vi "Find and Disable Selected Opposing Channels.vi"(8 "error in (no error)":errorcluster, 9 "Parent":string, 10 "Item Ref in":T1 format="%.0x", 11 "Tree":refnum<vi>) -> (0 "error out":errorcluster, 2 "Item Ref out":T1 format="%.0x", 3 "Tree Out":refnum<vi>)   [LabVIEW 2013, in "J1939 Addon System Explorer.lvlib"]
uses:
  J1939 Addon System Explorer.lvlib
  <vilib>/NI Veristand/Custom Device API/Custom Device Item Ref.ctl
  <vilib>/NI Veristand/Custom Device Tools/Custom Device Utility Library/Search Direction.ctl
  Shared/SubVIs/Constants.vi
  <vilib>/NI Veristand/Custom Device Tools/Custom Device Utility Library/Custom Device Utility Library.lvlib
  Shared/J1939 Addon Shared.lvlib
  <vilib>/NI Veristand/Custom Device API/Custom Device API.lvlib
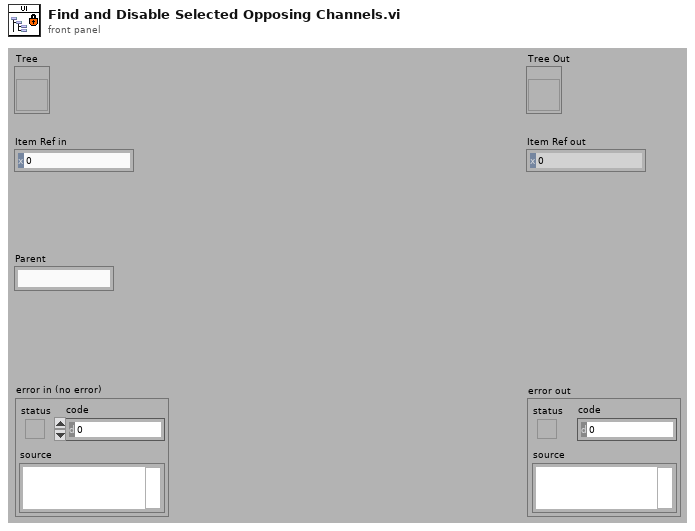
[diagram p1: front panel]
types:
  T1 = typedef "Custom Device API.lvlib/Custom Device Item Ref.ctl" = u64
  T2 = typedef "Custom Device Utility Library.lvlib/Search Direction.ctl" = enum16{"Down", "Up"}
  T3 = typedef "Custom Device API.lvlib/Custom Device Item Info.ctl" = cluster{"Name":string, "Is Channel":bool, "GUID":string, "Is Waveform":bool}
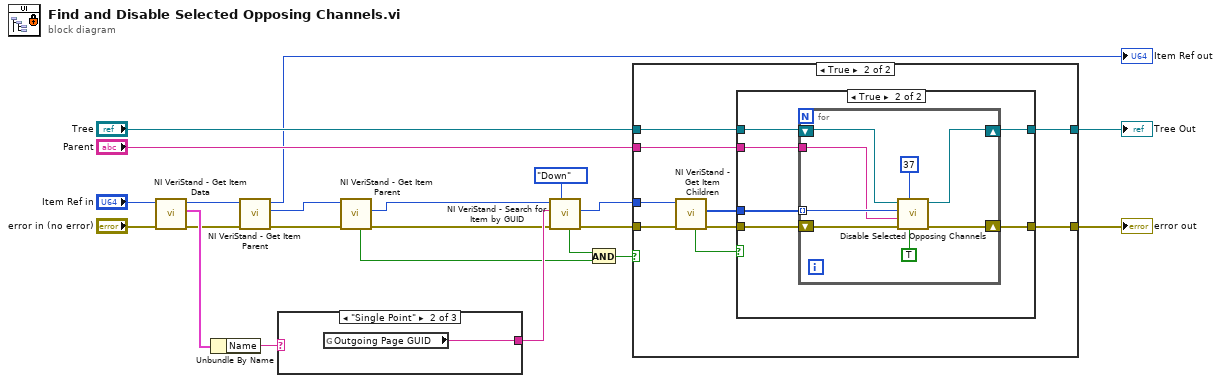
[diagram p0: block diagram]
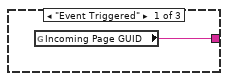
[diagram p4: hidden frame]
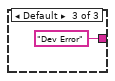
[diagram p5: hidden frame]
diagram:
  n1 = call <vilib>:"NI VeriStand - Get Item Data.vi"("error in (no error)"="error in (no error)", "Item Ref in"="Item Ref in") -> ("error out"=w8:errorcluster, "Item Info"=w21:T3, "Item Ref out"=w7:T1)  [unwired: 7 out]
  n2 = Unbundle By Name(w21) -> ("Name"=w22:string)
  n3 = call <vilib>:"NI VeriStand - Get Item Parent.vi"("error in (no error)"=w8, "Item Ref in"=w7) -> ("error out"=w6:errorcluster, "Parent Ref"=w5:T1, "Item Ref out"=→"Item Ref out":T1)  [unwired: 6 in, 1 out]
  n4 = case shown="\"Single Point\"" w22 {
    tunnel: [w23 w24 "Dev Error" ("Outgoing Page GUID")] -> w17
    frame "Event Triggered" {
      n5 = global read "Constants.vi" "Incoming Page GUID"() -> (w23:string)
    }
    frame "Single Point" {
      n6 = global read "Constants.vi" "Outgoing Page GUID"() -> (w24:string)
    }
    frame Default {
    }
  }
  n7 = call <vilib>:"NI VeriStand - Get Item Parent.vi"("error in (no error)"=w6, "Item Ref in"=w5) -> ("error out"=w4:errorcluster, "Parent Ref"=w3:T1, "Found"=w2:bool)  [unwired: 6 in, 1 out]
  n8 = call <vilib>:"NI VeriStand - Search for Item by GUID.vi"("Direction (Down)"=Search_Direction."Down", "error in"=w4, "Item GUID"=w17, "Section Ref in"=w3) -> ("error out"=w14:errorcluster, "Item Ref"=w9:T1, "Found"=w16:bool)  [unwired: 4 in, 1 out]
  n9 = And(x=w16, y=w2) -> (x .and. y?=w15:bool)
  n10 = case shown="True" w15 {
    tunnel: w9 -> [_ w32]
    tunnel: w14 -> [w27 w31]
    tunnel: [w27 w36] -> w11
    tunnel: "Tree" -> [w26 w35]
    tunnel: [w26 w34] -> w12
    tunnel: "Parent" -> [_ w33]
    frame False {
    }
    frame True {
      n11 = call <vilib>:"NI VeriStand - Get Item Children.vi"("error in (no error)"=w31, "Item Ref in"=w32) -> ("error out"=w30:errorcluster, "Child Refs"=w29:T1[], "Found"=w28:bool)  [unwired: 6 in, 1 out]
      n12 = case shown="True" w28 {
        tunnel: [w37 w44] -> w36
        tunnel: w35 -> [w38 w43]
        tunnel: [w38 w42] -> w34
        tunnel: w33 -> [_ w41]
        tunnel: w30 -> [w37 w40]
        tunnel: w29 -> [_ w39]
        frame False {
        }
        frame True {
          n13 = for {
            tunnel: w39 -> [w51] mode=indexing
            tunnel: w41 -> [w45]
            shift-right: [w48] -> w44
            shift-left: w40 -> [w49]
            shift-right: [w46] -> w42
            shift-left: w43 -> [w47]
            n14 = call "Disable Selected Opposing Channels.vi"("Disabled? (False)"=TRUE, "Symbol Index (38)"=37 ("Active Item:Symbol Index"), "error in (no error)"=w49, "Parent"=w45, "Node Ptr"=w51, "Tree"=w47) -> ("error out"=w48:errorcluster, "Tree Out"=w46:refnum<vi>)  [unwired: 3 in, 1 out]
          }
        }
      }
    }
  }
  "Tree Out" <- w12
  "error out" <- w11
